vi "FlatToRichgoogle_protobuf_SourceContext.vi"(5 "OutputClusterType":T1, 11 "InputCluster":T2) -> (3 "OutputCluster":T1)   [LabVIEW 2020, in "MeasurementLink Measurement Server Internal.lvlib"]
uses:
  MeasurementLink Measurement Server Internal.lvlib
  google_protobuf_SourceContext_Flat.ctl
  google_protobuf_SourceContext.ctl
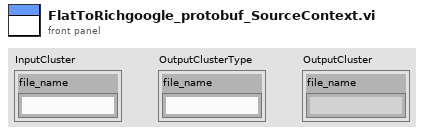
[diagram p1: front panel]
types:
  T1 = typedef "MeasurementLink Measurement Server Internal.lvlib/google_protobuf_SourceContext.ctl" = cluster{"file_name":string}
  T2 = typedef "MeasurementLink Measurement Server Internal.lvlib/google_protobuf_SourceContext_Flat.ctl" = cluster{"file_name":string}
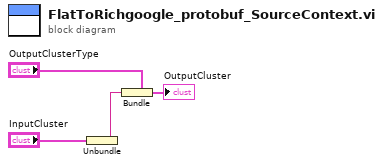
[diagram p0: block diagram]
diagram:
  n1 = Unbundle "Unbundle"("InputCluster") -> ("file_name"=w1:string)
  n2 = Bundle "Bundle"(cluster="OutputClusterType", "file_name"=w1) -> (→"OutputCluster":T1)
